vi "Test Coffee Shop Removed Customer is Cleared.vi"(8 "error in (no error)":errorcluster, 11 "Coffee Shop Test In":refnum<class "Coffee Shop Test.lvclass">) -> (0 "error out":errorcluster, 3 "Coffee Shop Test Out":refnum<class "Coffee Shop Test.lvclass">)   [LabVIEW 2020, in "Coffee Shop Test.lvclass"]
uses:
  Coffee Shop Test.lvclass
  Coffee Shop/Coffee Shop.lvclass
  <vilib>/Asteme/Triarc Framework/Process/Process.lvclass
  C:/Program Files (x86)/National Instruments/LabVIEW 2020/vi.lib/Asteme/Triarc Framework/Application/Application.lvclass
  C:/Program Files (x86)/National Instruments/LabVIEW 2020/vi.lib/Asteme/Triarc Framework/Process/Process.lvclass
  C:/Program Files (x86)/National Instruments/LabVIEW 2020/vi.lib/Asteme/Triarc Framework/Base/Base.lvclass
  C:/Program Files (x86)/National Instruments/LabVIEW 2020/vi.lib/Asteme/Triarc Framework/Error Handler Interface/Error Handler Interface.lvclass
  C:/Program Files (x86)/National Instruments/LabVIEW 2020/vi.lib/Asteme/Triarc Framework/Logging/Logging.lvclass
  C:/Users/anton/Documents/GitHub/Triarc-Examples/Coffee Shop/Coffee Shop/Coffee Shop.lvclass
  <vilib>/Asteme/Triarc Framework/Application/Application.lvclass
  <vilib>/Asteme/Triarc Framework/Process/Public/Lifecycle/Lifecycle State.ctl
  <vilib>/Asteme/LUnit/Test Case.lvclass
  C:/Program Files (x86)/National Instruments/LabVIEW 2020/vi.lib/Asteme/Triarc Framework Test Suite/Application Test/Application Test.lvclass
  C:/Program Files (x86)/National Instruments/LabVIEW 2020/vi.lib/Asteme/Triarc Framework Test Suite/Process Test/Process Test.lvclass
  C:/Program Files (x86)/National Instruments/LabVIEW 2020/vi.lib/Asteme/Triarc Framework Test Suite/Base Class Test/Base Test.lvclass
  C:/Program Files (x86)/National Instruments/LabVIEW 2020/vi.lib/Asteme/LUnit/Test Case.lvclass
  C:/Users/anton/Documents/GitHub/Triarc-Examples/Coffee Shop/Coffee Shop Test/Coffee Shop Test.lvclass
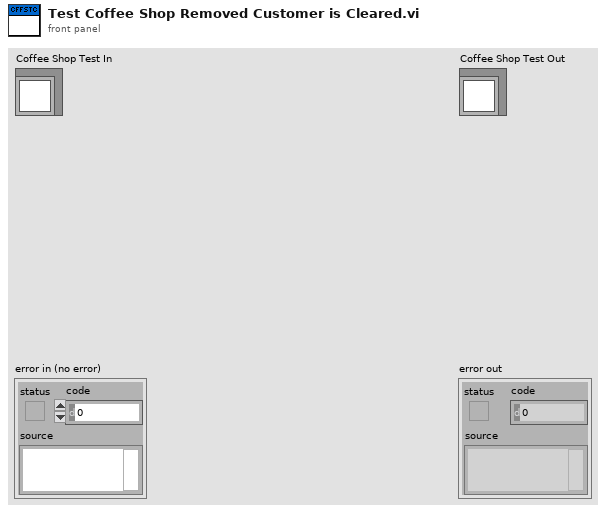
[diagram p1: front panel]
types:
  T1 = typedef "TF.lvlib/Process.lvclass/Lifecycle State.ctl" = enum16{"Uninitialized", "Initialized", "Started", "Running", "Stopped", "Finished"}
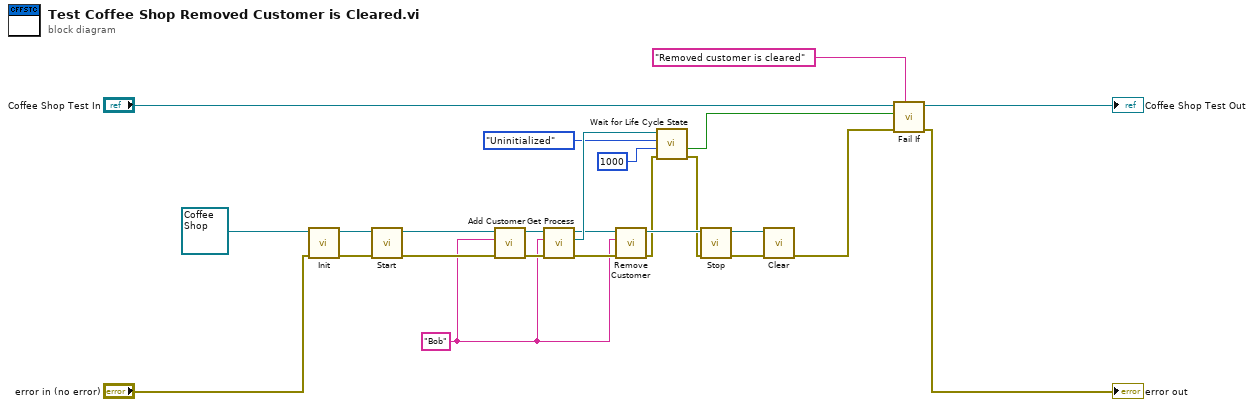
[diagram p0: block diagram]
diagram:
  w6 = "Bob" ("Name")
  n1 = call-dynamic "Init.vi"("error in (no error)"="error in (no error)", "Process In"=refnum<class "Coffee Shop.lvclass"> refnum ("Coffee Shop.lvclass")) -> ("error out"=w23:errorcluster, "Process Out"=w24:refnum<class "Coffee Shop.lvclass">)  [unwired: 8 in]
  n2 = call <vilib>:"Start.vi"("error in (no error)"=w23, "Process In"=w24) -> ("error out"=w18:errorcluster, "Process Out"=w17:refnum<class "Coffee Shop.lvclass">)  [unwired: 8 in]
  n3 = call "Add Customer.vi"("error in (no error)"=w18, "Name"=w6, "Coffee Shop in"=w17) -> ("error out"=w19:errorcluster, "Coffee Shop out"=w10:refnum<class "Coffee Shop.lvclass">)  [unwired: 7 in]
  n4 = call <vilib>:"Get Process.vi"("error in (no error)"=w19, "Process Name"=w6, "Rig In"=w10) -> ("error out"=w11:errorcluster, "App Process"=w9:refnum<class "Process.lvclass">, "Rig Out"=w8:refnum<class "Coffee Shop.lvclass">)  [unwired: 6 in]
  n5 = call "Remove Customer.vi"("error in (no error)"=w11, "Name"=w6, "Coffee Shop In"=w8) -> ("error out"=w5:errorcluster, "Coffee Shop Out"=w7:refnum<class "Coffee Shop.lvclass">)  [unwired: 7 in]
  n6 = call <vilib>:"Wait for Life Cycle State.vi"("error in (no error)"=w5, "timeout in ms (-1)"=1000, "Lifecycle State"=Lifecycle_State."Uninitialized", "Process In"=w9) -> ("error out"=w4:errorcluster, "timed out?"=w1:bool)  [unwired: 5 in, 1 out]
  n7 = call <vilib>:"Stop.vi"("error in (no error)"=w4, "Process In"=w7) -> ("error out"=w21:errorcluster, "Process Out"=w22:refnum<class "Coffee Shop.lvclass">)  [unwired: 7 in, 1 out]
  n8 = call-dynamic "Clear.vi"("error in (no error)"=w21, "Application In"=w22) -> ("error out"=w14:errorcluster)  [unwired: 9 in]
  n9 = call <vilib>:"Fail If.vi"("Description"="Removed customer is cleared", "error in (no error)"=w14, "Fail?"=w1, "Test Case In"="Coffee Shop Test In") -> ("error out"=→"error out":errorcluster, "Test Case Out"=→"Coffee Shop Test Out":refnum<class "Coffee Shop Test.lvclass">)  [unwired: 6 in]
